vi "New Formatted String Binding.vi"(7 "Format String":string, 10 "Str Refnum":refnum<vi>) -> (0 "error out":errorcluster, 3 "FormattedStringBinding":refnum<class "FormattedStringBinding.lvclass">)   [LabVIEW 2015, in "Transport.lvlib" / "FormattedStringBinding.lvclass"]
doc: "<License>\nCopyright © 2017 Composed Systems, LLC | All rights reserved\nwww.composed.io\n\nAuthor: Ethan Stern <ethan.stern@composed.io>\n\nThis software is provided \"AS IS\" WITHOUT WARRANTIES, either express or implied, AND IS FOR EDUCATIONAL PURPOSES ONLY.\n</License>"
uses:
  FormattedStringBinding.lvclass
  FormattedStringBinding.lvclass/FormattedStringBinding.ctl
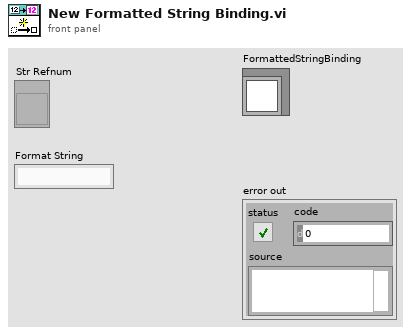
[diagram p1: front panel]
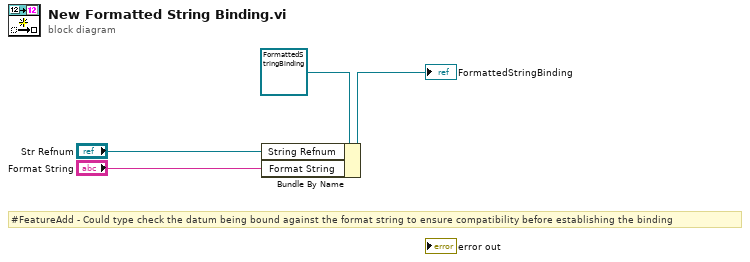
[diagram p0: block diagram]
diagram:
  # "#FeatureAdd - Could type check the datum being bound against the format string to ensure compatibility before establishing the binding"
  n1 = Bundle By Name(cluster=refnum<class "FormattedStringBinding.lvclass"> refnum ("TerminalBinding in"), "String Refnum"="Str Refnum", "Format String"="Format String") -> (→"FormattedStringBinding":refnum<class "FormattedStringBinding.lvclass">)
